vi "Skyline Send Waveform File.vi"(8 "error in":errorcluster, 9 "properties":cluster{"Key":string, "Value":string}[](array[cluster]) caption="properties (null)", 11 "data in":waveform(dbl)[](array[waveform])) -> (0 "error out":errorcluster, 2 "size in bytes":i32, 3 "file id":string)   [LabVIEW 2019]
uses:
  <vilib>/Skyline/File/File/NI Skyline File.lvclass
  <vilib>/Skyline/File/File/Send Buffer.vi
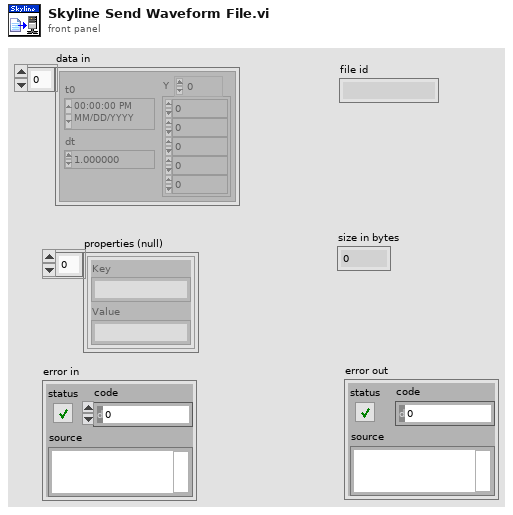
[diagram p1: front panel]
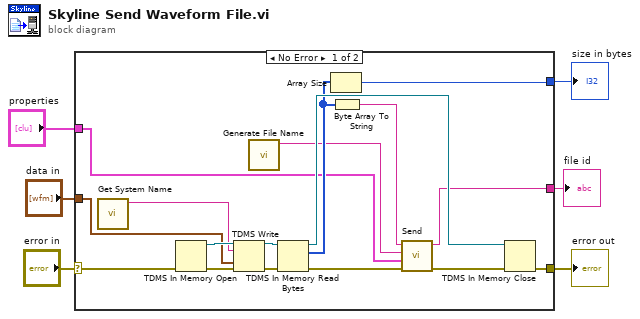
[diagram p0: block diagram]
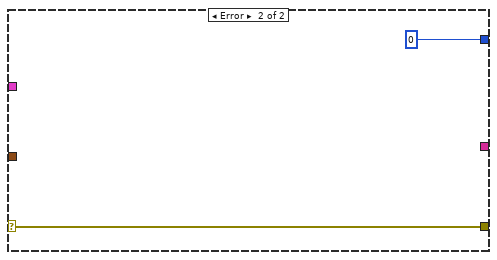
[diagram p2: hidden frame]
diagram:
  n1 = case shown="No Error" "error in" {
    selector: "error in" -> [w16 w25]
    tunnel: [w18 w25] -> w6
    tunnel: "properties" -> [w12 _]
    tunnel: "data in" -> [w22 _]
    tunnel: [w14 0] -> w2
    tunnel: [w7 _] -> w1
    frame No Error {
      n2 = call "Get System Name.vi"() -> ("name"=w13:string)  [unwired: 11 in]
      n3 = TDMS In Memory Open(8:w16) -> (0:w17:errorcluster, 3:w23:refnum<k34>)  [unwired: 1 in]
      n4 = TDMS Write(0:w23, 5:w13, 9:w22, 11:w17) -> (4:w20:refnum<k34>, 15:w21:errorcluster)  [unwired: 2 in, 2 out]
      n5 = call "Generate File Name.vi"() -> ("file name"=w10:string)  [unwired: 11 in]
      n6 = TDMS In Memory Read Bytes(8:w21, 11:w20) -> (0:w11:errorcluster, 2:w15:u8[], 3:w19:refnum<k34>)  [unwired: 2 in]
      n7 = Array Size(array=w15) -> (size(s)=w14:i32)
      n8 = Byte Array To String(unsigned byte array=w15) -> (string=w9:string)
      n9 = call-poly <vilib>:"Send.vi"("error in (no error)"=w11, "properties"=w12, "file name"=w10, "data"=w9) -> ("error out"=w8:errorcluster, "id"=w7:string)  [unwired: 5 in]
      n10 = TDMS In Memory Close(8:w8, 11:w19) -> (0:w18:errorcluster)  [unwired: 2 in]
    }
    frame Error {
    }
  }
  "error out" <- w6
  "size in bytes" <- w2
  "file id" <- w1
